vi "Compressor Begin.vi"(1 "error in (no error)":errorcluster) -> (0 "error out":errorcluster)   [LabVIEW 2014]
uses:
  <vilib>/Rock Robotics/WPI/Compressor/WPI_CompressorGetSetRefNum.vi
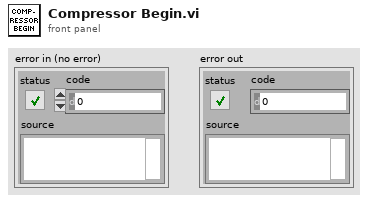
[diagram p1: front panel]
types:
  T1 = typedef "WPI_CompressorDevRef.ctl" = cluster{"DevStatus":errorcluster, "Pneumatics Control Module":u8}
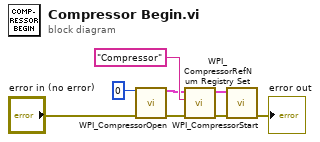
[diagram p0: block diagram]
diagram:
  n1 = call <vilib>:"WPI_CompressorOpen.vi"("Pneumatics Control Module (0)"=u8 0, "error in (no error)"="error in (no error)") -> ("CompressorDevRef"=w3:T1, "error out"=w5:errorcluster)  [unwired: 12 in]
  n2 = call <vilib>:"WPI_CompressorRefNum Registry Set.vi"("error in (no error)"=w5, "refnum name"="Compressor", "CompressorDevRef"=w3) -> ("error out"=w7:errorcluster, "CompressorDevRef"=w6:T1)  [unwired: 7 in]
  n3 = call <vilib>:"WPI_CompressorStart.vi"("error in (no error)"=w7, "CompressorDevRef"=w6) -> ("error out"=→"error out":errorcluster)  [unwired: 8 in, 1 out]
